vi "p1.vi"() -> ()   [LabVIEW 2025, in "d12.lvlib"]
uses:
  d12.lvlib
  lv2025-aoc/AOC/AOC.lvlib
panel:
  out "Answer":u64=7670
  in  "Example":string="???.### 1,1,3\n.??..??...?##. 1,1,3\n?#?#?#?#?#?#?#? 1,3,1,6\n????.#...#... 4,1,1\n????.######..#####. 1,6,5\n?###???????? 3,2,1"
  in  "Example":bool
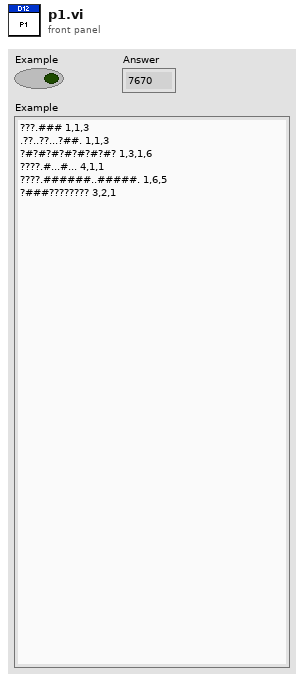
[diagram p1: front panel]
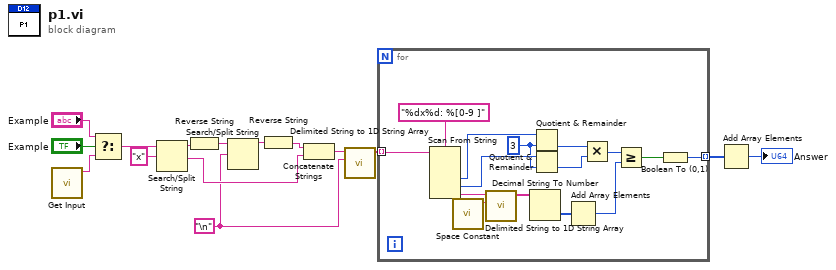
[diagram p0: block diagram]
diagram:
  w3 = "\n"
  n1 = call "Get Input.vi"() -> ("Input"=w15:string)  [unwired: 11 in]
  n2 = Select(t="Example", s="Example", f=w15) -> (s? t:f=w11:string)
  n3 = Search/Split String(string=w11, search string/char (-)="x") -> (substring before match=w9:string, match + rest of string=w5:string)  [unwired: 1 in, 1 out]
  n4 = Reverse String(1:w9) -> (0:w8:string)
  n5 = Search/Split String(string=w8, search string/char (-)=w3) -> (substring before match=w7:string)  [unwired: 1 in, 2 out]
  n6 = Reverse String(1:w7) -> (0:w6:string)
  n7 = Concatenate Strings(w6, w5) -> (w4:string)
  n8 = call <vilib>:"Delimited String to 1D String Array.vi"("delimiter"=w3, "delimited string"=w4) -> ("string array"=w2:string[])  [unwired: 9 in]
  n9 = for {
    tunnel: w2 -> [w30] mode=indexing
    tunnel: [w16] -> w1 mode=indexing
    w23 = 3 ("y")
    n10 = Scan From String(format string="%dx%d: %[0-9 ]", input string=w30) -> (output 1=w25:i32, output 2=w24:i32, output 3=w28:string)  [unwired: 5 in, 3 out]
    n11 = call <vilib>:"Space Constant.vi"() -> ("String"=w27:string)
    n12 = call <vilib>:"Delimited String to 1D String Array.vi"("delimiter"=w27, "delimited string"=w28) -> ("string array"=w26:string[])  [unwired: 9 in]
    n13 = Decimal String To Number(string=w26) -> (number=w22:i32[])  [unwired: 2 in, 1 out]
    n14 = Quotient & Remainder(x=w25, y=w23) -> (floor(x/y)=w21:i32)  [unwired: 1 out]
    n15 = Quotient & Remainder(x=w24, y=w23) -> (floor(x/y)=w20:i32)  [unwired: 1 out]
    n16 = Add Array Elements(numeric array=w22) -> (sum=w18:i32)
    n17 = Multiply(x=w21, y=w20) -> (x*y=w19:i32)
    n18 = Greater Or Equal?(x=w19, y=w18) -> (x >= y?=w17:bool)
    n19 = Boolean To (0,1)(Boolean=w17) -> (0, 1=w16:i16)
  }
  n20 = Add Array Elements(numeric array=w1) -> (sum=→"Answer":i16)
